vi "Get ClassID and ClassName Table(冲突时的文件备份2013-03-27 14-09-21).vi"(8 "错误输入（无错误）":errorcluster) -> (0 "错误输出":errorcluster, 3 "ClassID and ClassName":string[][](table))   [LabVIEW 2012, in "Application.lvlib"]
uses:
  Application.lvlib
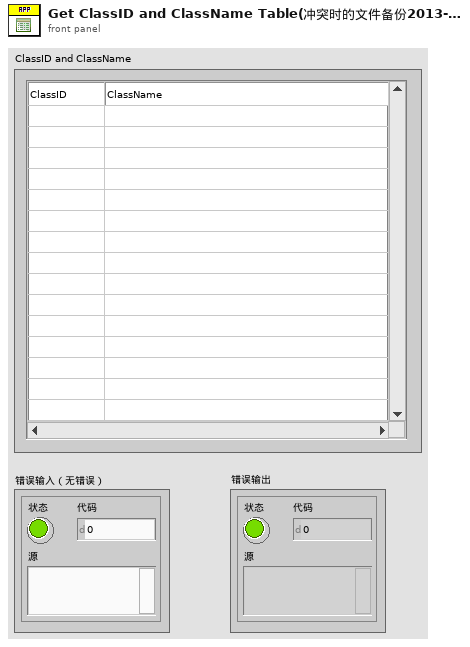
[diagram p1: front panel]
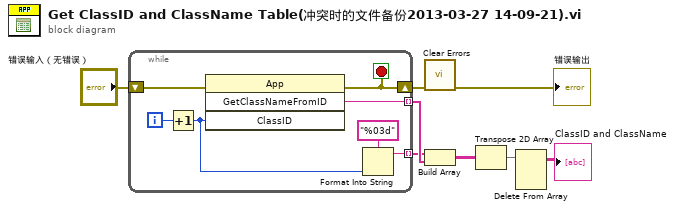
[diagram p0: block diagram]
diagram:
  n1 = while {
    tunnel: [w14] -> w8 mode=indexing
    tunnel: [w11] -> w6 mode=indexing
    shift-right: [w9] -> w4
    shift-left: "错误输入（无错误）" -> [w10]
    i -> [w15]
    stop <- w9 stop-if-true
    n2 = Increment(x=w15) -> (x+1=w12:i32)
    n3 = invoke class="App" method="GetClassNameFromID"(error in=w10, "ClassID"=w12) -> (error out=w9:errorcluster, "GetClassNameFromID"=w14:string)  [unwired: 2 in, 2 out]
    n4 = Format Into String(format string="%03d" ("格式字符串"), w12) -> (resulting string=w11:string)  [unwired: 2 in, 1 out]
  }
  n5 = call <vilib>:"Clear Errors.vi"("error in (no error)"=w4) -> ("error out"=→"错误输出":errorcluster)  [unwired: 6 in]
  n6 = Build Array(w6, w8) -> (w7:string[][])
  n7 = Transpose 2D Array(2D array=w7) -> (transposed array=w2:string[][])
  n8 = Delete From Array(array=w2) -> (array with subset deleted=→"ClassID and ClassName":string[][])  [unwired: 3 in, 1 out]
